vi "SettingsDialog.vi"(10 "TreeSettings In":T1, 11 "Settings In":T2) -> (2 "TreeSettings Out":T1, 3 "Settings Out":T2)   [LabVIEW 2011, in "VariantXControl__VP.xctl"]
doc: "This will show the Variant Tree Settings dialog."
uses:
  VariantXControl__VP.xctl
  Permissions.ctl
  TreeSettings.ctl
  <vilib>/event_ctls.llb/eventvkey.ctl
panel:
  in  "Colorize.Active":bool
  in  "Traverse.Active":bool
  in  "Colorize":bool
  in  "Traverse Attributes":bool
  in  "Resettable":bool
  in  "OK":bool
  out "Status Bar":string
  # "User\npermissions"
  # "Status"
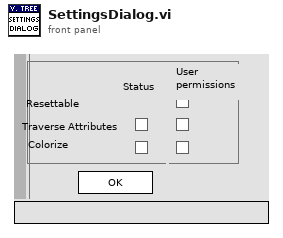
[diagram p1: front panel]
types:
  T1 = typedef "VariantXControl__VP.xctl/TreeSettings.ctl" = cluster{"Traverse":bool, "Colorize":bool}
  T2 = typedef "VariantXControl__VP.xctl/Permissions.ctl" = cluster{"Reset":bool, "TraverseAttributes":bool, "Colorize":bool}
  T3 = typedef "eventvkey.ctl" = enum16{"ASCII", "Enter", "Return", "Shift", "Ctrl", "Alt", "Cmd", "Opt", "Caps", "NumLock", "Clear", "Break", "Up", "Down", "Left", "Right", "Insert", "Delete", "Home", "End", "PageUp", "PageDown", "Escape", "Help", "Pause", "ScrollLock", "F1", "F2", "F3", "F4", "F5", "F6", "F7", "F8", "F9", "F10", "F11", "F12", "F13", "F14", "F15", "F16", "F17", "F18", "F19", "F20", "F21", "F22", "F23", "F24", "Play", "VolumeUp", "VolumeDown", "Mute", "Two Byte Char"}
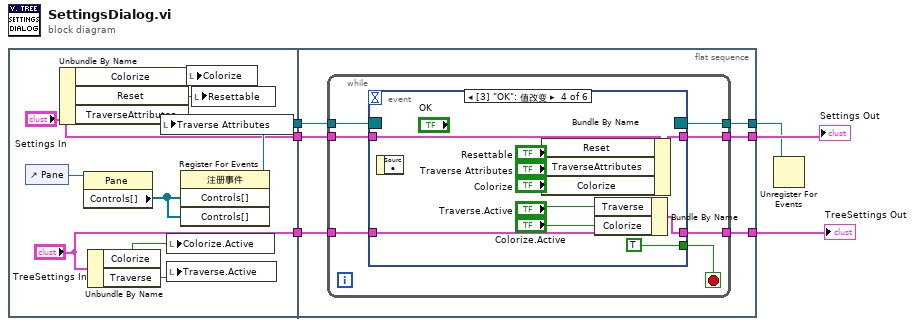
[diagram p0: block diagram]
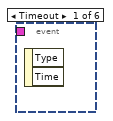
[diagram p2: hidden frame]
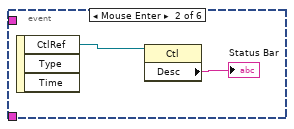
[diagram p3: hidden frame]
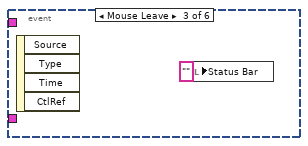
[diagram p4: hidden frame]
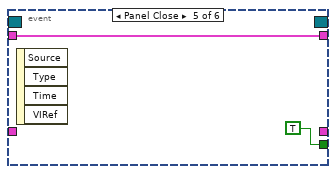
[diagram p5: hidden frame]
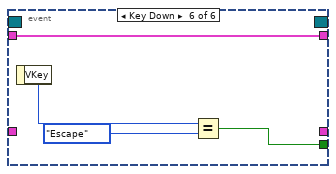
[diagram p6: hidden frame]
diagram:
  n1 = flat-sequence {
    tunnel: [w14] -> w6
    tunnel: ["Settings In"] -> w5
    tunnel: ["TreeSettings In"] -> w2
    tunnel: w6 -> [w22]
    tunnel: w5 -> [w21]
    tunnel: [w20] -> w4
    tunnel: [w19] -> w3
    tunnel: w2 -> [w18]
    tunnel: [w17] -> w1
    frame #0 {
      n2 = control-ref of="Pane"() -> (w15:refnum<vi>)
      n3 = Unbundle By Name("Settings In") -> ("Colorize"=w11:bool, "Reset"=w16:bool, "TraverseAttributes"=w12:bool)
      n4 = property class="Pane"(reference=w15) -> ("Controls[]"=w9:refnum<vi>[])  [unwired: 1 in, 2 out]
      n5 = Unbundle By Name("TreeSettings In") -> ("Colorize"=w8:bool, "Traverse"=w10:bool)
      n6 = local write "Traverse Attributes"(w12) -> ()
      n7 = local write "Colorize.Active"(w8) -> ()
      n8 = local write "Traverse.Active"(w10) -> ()
      n9 = register-events(w9, w9) -> (reference out=w14:refnum<event-registration>)  [unwired: 2 in, 1 out]
      n10 = local write "Colorize"(w11) -> ()
      n11 = local write "Resettable"(w16) -> ()
    }
    frame #1 {
      n12 = while {
        tunnel: w22 -> [w29]
        tunnel: w21 -> [w28]
        tunnel: [w27] -> w20
        tunnel: [w25] -> w19
        tunnel: w18 -> [w24]
        tunnel: [w23] -> w17
        stop <- w26 stop-if-true
        n13 = event shown="[3] \"OK\": 值改变" {
          selector: w29 -> [_ _ _ _ _ _]
          dyn-events: [_ _ _ _ _ _] -> w25
          timeout: _ -> [_ _ _ _ _ _]
          tunnel: w28 -> [_ _ _ w42 w43 w48]
          tunnel: [_ _ _ w41 w43 w48] -> w27
          tunnel: [_ _ _ TRUE TRUE w45] -> w26
          tunnel: w24 -> [_ _ _ w36 _ _]
          tunnel: [_ _ _ w35 _ _] -> w23
          event Timeout {
            n14 = event-data() -> ()  [unwired: 1 in, 2 out]
          }
          event Mouse Enter {
            n15 = event-data() -> ("CtlRef"=w31:refnum<vi>)  [unwired: 1 in, 2 out]
            n16 = property class="Ctl"(reference=w31) -> ("Desc"=→"Status Bar":string)  [unwired: 1 in, 2 out]
          }
          event Mouse Leave {
            n17 = event-data() -> ()  [unwired: 1 in, 4 out]
            n18 = local write "Status Bar"("" ("Status Bar")) -> ()
          }
          event "OK": Value Change {
            n19 = event-data() -> ()  [unwired: 1 in, 1 out]
            n20 = Bundle By Name(cluster=w42, "Reset"="Resettable", "TraverseAttributes"="Traverse Attributes", "Colorize"="Colorize") -> (w41:T2)
            n21 = Bundle By Name(cluster=w36, "Traverse"="Traverse.Active", "Colorize"="Colorize.Active") -> (w35:T1)
          }
          event Panel Close {
            n22 = event-data() -> ()  [unwired: 1 in, 4 out]
          }
          event Key Down {
            n23 = event-data() -> ("VKey"=w47:T3)  [unwired: 1 in]
            n24 = Equal?(x=w47, y=eventvkey."Escape") -> (x = y?=w45:bool)
          }
        }
      }
    }
  }
  n25 = Unregister For Events(event registration refnum=w3) -> ()  [unwired: 1 in, 1 out]
  "Settings Out" <- w4
  "TreeSettings Out" <- w1
